vi "TDT ET-Check for Errors.vi"(0 "TCP":T1, 7 "TCP return value":i32, 9 "Command":string, 11 "error in (no error)":errorcluster) -> (4 "TCP Thru":T1, 15 "error out":errorcluster)   [LabVIEW 2020]
uses:
  Utility VIs/Type Defs/TCP Params.ctl
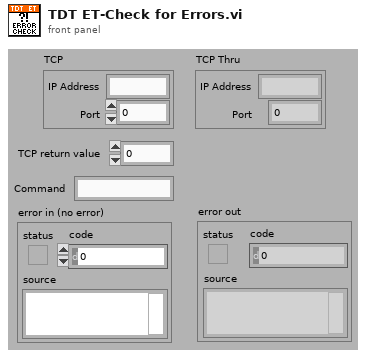
[diagram p1: front panel]
types:
  T1 = typedef "TCP Params.ctl" = cluster{"IP Address":string, "Port":i32}
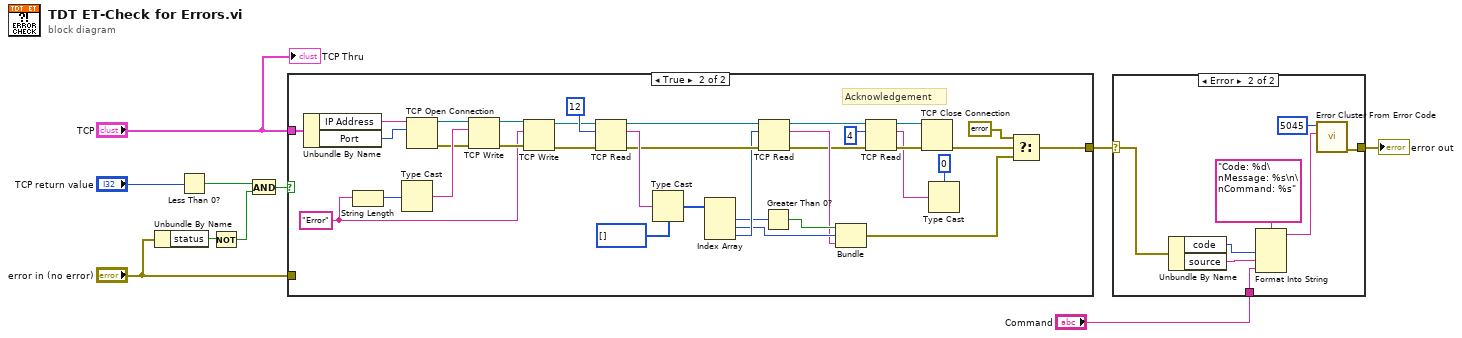
[diagram p0: block diagram]
diagram:
  n1 = Unbundle By Name("error in (no error)") -> ("status"=w7:bool)
  n2 = Less Than 0?(x="TCP return value") -> (x < 0?=w9:bool)
  n3 = Not(x=w7) -> (.not. x?=w6:bool)
  n4 = And(x=w9, y=w6) -> (x .and. y?=w8:bool)
  n5 = case shown="True" w8 {
    tunnel: "TCP" -> [_ w34]
    tunnel: [w11 w12] -> w3
    tunnel: "error in (no error)" -> [w11 _]
    frame False {
    }
    frame True {
      w31 = "Error" ("string")
      # "Acknowledgement"
      n6 = Unbundle By Name(w34) -> ("IP Address"=w44:string, "Port"=w45:i32)
      n7 = String Length(string=w31) -> (length=w36:i32)
      n8 = Type Cast(x=w36) -> (*(type *) &x=w35:string)  [unwired: 1 in]
      n9 = TCP Open Connection(address=w44, remote port or service name=w45) -> (connection ID=w33:refnum<k5>, error out=w32:errorcluster)  [unwired: 3 in]
      n10 = TCP Write(connection ID=w33, data in=w35, error in (no error)=w32) -> (connection ID out=w37:refnum<k5>, error out=w43:errorcluster)  [unwired: 1 in, 1 out]
      n11 = TCP Write(connection ID=w37, data in=w31, error in (no error)=w43) -> (connection ID out=w28:refnum<k5>, error out=w29:errorcluster)  [unwired: 1 in, 1 out]
      n12 = TCP Read(connection ID=w28, bytes to read=12, error in (no error)=w29) -> (connection ID out=w23:refnum<k5>, data out=w26:string, error out=w24:errorcluster)  [unwired: 2 in]
      n13 = Type Cast(type=i32[] [], x=w26) -> (*(type *) &x=w25:i32[])
      n14 = Index Array(array=w25) -> (element #1=w21:i32, element #2=w19:i32, element #3=w22:i32)  [unwired: 3 in]
      n15 = TCP Read(connection ID=w23, bytes to read=w22, error in (no error)=w24) -> (connection ID out=w16:refnum<k5>, data out=w18:string, error out=w17:errorcluster)  [unwired: 2 in]
      n16 = Greater Than 0?(x=w21) -> (x > 0?=w20:bool)
      n17 = Bundle(w20, w19, "data out"=w18) -> (w14:cluster{bool, i32, "data out":string})  [unwired: 1 in]
      n18 = TCP Read(connection ID=w16, bytes to read=4, error in (no error)=w17) -> (connection ID out=w40:refnum<k5>, data out=w39:string, error out=w41:errorcluster)  [unwired: 2 in]
      n19 = TCP Close Connection(connection ID=w40, error in (no error)=w41) -> (error out=w15:errorcluster)  [unwired: 1 in, 1 out]
      n20 = Type Cast(type=0, x=w39) -> ()  [unwired: 1 out]
      n21 = Select(t=cluster{bool, i32, "data out":string} {FALSE, 0, "data out"=""}, s=w15, f=w14) -> (s? t:f=w12:cluster{bool, i32, "data out":string})
    }
  }
  n22 = case shown="Error" w3 {
    selector: w3 -> [w46 w50]
    tunnel: [w46 w54] -> w2
    tunnel: "Command" -> [_ w47]
    frame No Error {
    }
    frame Error {
      n23 = Unbundle By Name(w50) -> ("code"=w49:i32, "source"=w48:string)
      n24 = Format Into String(format string="Code: %d\nMessage: %s\n\nCommand: %s", w49, w48, w47) -> (resulting string=w52:string)  [unwired: 2 in, 1 out]
      n25 = call <vilib>:"Error Cluster From Error Code.vi"("error message (\"\")"=w52, "error code (0)"=5045) -> ("error out"=w54:errorcluster)  [unwired: 7 in]
    }
  }
  "error out" <- w2
  "TCP Thru" <- "TCP"
